vi "FindTabPageByName.vi"(10 "Name":string, 11 "Tab Control":refnum<vi>) -> (2 "found?":bool, 3 "Page Refnum":refnum<vi>)   [LabVIEW 2017]
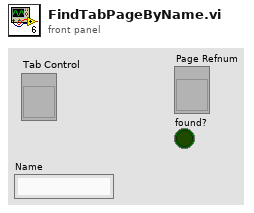
[diagram p1: front panel]
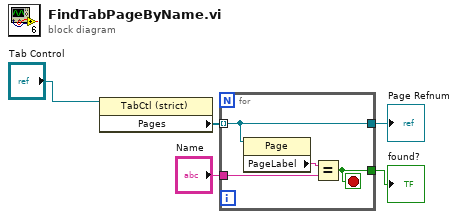
[diagram p0: block diagram]
diagram:
  n1 = property class="TabCtl (strict)"(reference="Tab Control") -> ("Pages"=w5:refnum<vi>[])  [unwired: 1 in, 2 out]
  n2 = for {
    tunnel: w5 -> [w6] mode=indexing
    tunnel: "Name" -> [w8]
    tunnel: [w7] -> w2
    tunnel: [w6] -> w3
    stop <- w7 stop-if-true
    n3 = property class="Page"(reference=w6) -> ("PageLabel"=w9:string)  [unwired: 1 in, 2 out]
    n4 = Equal?(x=w9, y=w8) -> (x = y?=w7:bool)
  }
  "Page Refnum" <- w3
  "found?" <- w2
